vi "Check if autofocus.vi"(8 "error in (no error)":errorcluster, 10 "Message in":refnum<class "GenericMessage.lvclass">, 11 "StageSPIM in":refnum<class "StageSPIM.lvclass">) -> (0 "error out":errorcluster, 2 "Message out":refnum<class "GenericMessage.lvclass">, 3 "StageSPIM out":refnum<class "StageSPIM.lvclass">)   [LabVIEW 2012, in "StageSPIM.lvclass"]
uses:
  StageSPIM.lvclass
  <vilib>/Distrio/Murmex/GenericMessage/GenericMessage.lvclass
  StageSPIM.lvclass/StageSPIM.ctl
  <vilib>/Distrio/Murmex/Message/Message.lvclass
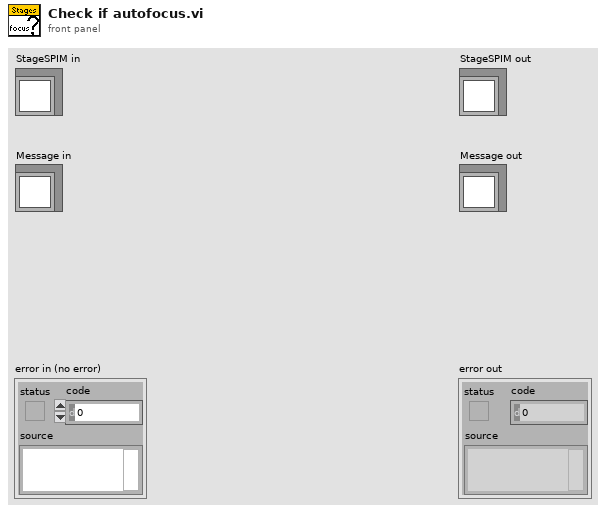
[diagram p1: front panel]
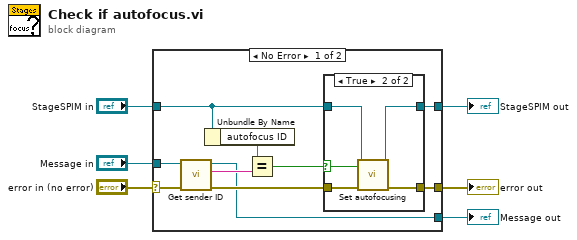
[diagram p0: block diagram]
diagram:
  n1 = case shown="No Error" "error in (no error)" {
    selector: "error in (no error)" -> [w15 w26]
    tunnel: [w9 w26] -> w5
    tunnel: [w8 w25] -> w3
    tunnel: "StageSPIM in" -> [w10 w25]
    tunnel: "Message in" -> [w16 w24]
    tunnel: [w7 w24] -> w1
    frame No Error {
      n2 = call <vilib>:"Get sender ID.vi"("error in (no error)"=w15, "Message in"=w16) -> ("error out"=w12:errorcluster, "sender"=w14:string, "Message out"=w7:refnum<class "GenericMessage.lvclass">)  [unwired: 7 in]
      n3 = Unbundle By Name(w10) -> ("autofocus ID"=w13:string)
      n4 = Equal?(x=w13, y=w14) -> (x = y?=w11:bool)
      n5 = case shown="True" w11 {
        selector: w11 -> [_ w22]
        tunnel: w12 -> [w17 w23]
        tunnel: w10 -> [w18 w21]
        tunnel: [w17 w20] -> w9
        tunnel: [w18 w19] -> w8
        frame False {
        }
        frame True {
          n6 = call-dynamic "Set autofocusing.vi"("error in (no error)"=w23, "autofocusing?"=w22, "StageSPIM in"=w21) -> ("error out"=w20:errorcluster, "StageSPIM out"=w19:refnum<class "StageSPIM.lvclass">)  [unwired: 7 in]
        }
      }
    }
    frame Error {
    }
  }
  "error out" <- w5
  "StageSPIM out" <- w3
  "Message out" <- w1
